vi "Register by Name.vi"(7 "Event":refnum<class "Event.lvclass">, 8 "error in (no error)":errorcluster, 9 "Event Fire Handler":refnum<class "Event Generated Msg.lvclass">, 10 "Sink Name":string, 11 "Event Source in":refnum<class "Event Source.lvclass">) -> (0 "error out":errorcluster, 3 "Event Source out":refnum<class "Event Source.lvclass">)   [LabVIEW 2016, in "Event Source.lvlib" / "Event Source.lvclass"]
uses:
  Event Source.lvclass
  Event/Event.lvclass
  Event Source Messages/Event Generated Msg/Event Generated Msg.lvclass
  Event Source.lvclass/Event Source.ctl
  <vilib>/ActorFramework/Message Enqueuer/Message Enqueuer.lvclass
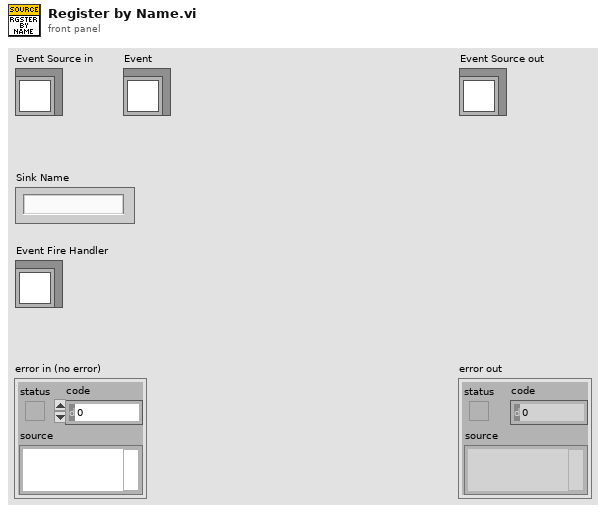
[diagram p1: front panel]
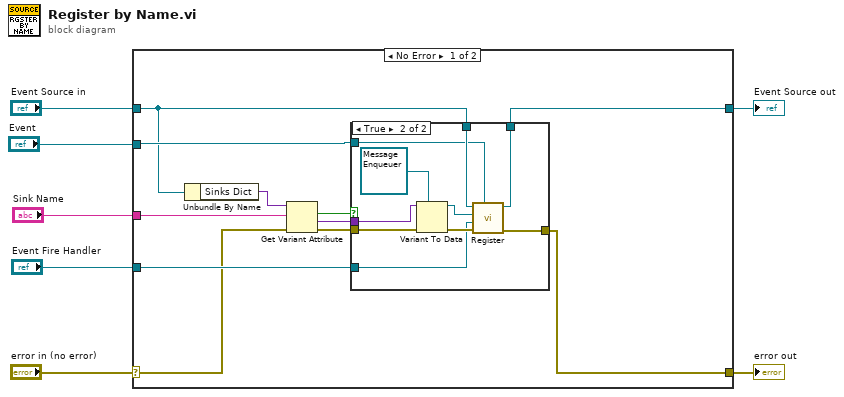
[diagram p0: block diagram]
diagram:
  n1 = case shown="No Error" "error in (no error)" {
    selector: "error in (no error)" -> [w9 w32]
    tunnel: [w8 w32] -> w6
    tunnel: [w10 w31] -> w4
    tunnel: "Event Source in" -> [w11 w31]
    tunnel: "Sink Name" -> [w17 _]
    tunnel: "Event Fire Handler" -> [w13 _]
    tunnel: "Event" -> [w12 _]
    frame No Error {
      n2 = Unbundle By Name(w11) -> ("Sinks Dict"=w18:variant)
      n3 = Get Variant Attribute(Variant=w18, name=w17, error in=w9) -> (found=w16:bool, value=w15:variant, error out=w14:errorcluster)  [unwired: 1 in, 1 out]
      n4 = case shown="True" w16 {
        tunnel: w15 -> [_ w28]
        tunnel: w14 -> [w20 w29]
        tunnel: w13 -> [_ w25]
        tunnel: w11 -> [w19 w24]
        tunnel: w12 -> [_ w23]
        tunnel: [w20 w22] -> w8
        tunnel: [w19 w21] -> w10
        frame False {
        }
        frame True {
          n5 = Variant To Data(error in=w29, type=refnum<class "Message Enqueuer.lvclass"> refnum ("Actor's Enqueuer"), Variant=w28) -> (data=w26:refnum<class "Message Enqueuer.lvclass">, error out=w27:errorcluster)
          n6 = call "Register.vi"("Event"=w23, "Error In"=w27, "Event Fire Handler"=w25, "Registrant Enq"=w26, "Event Source In"=w24) -> ("Error Out"=w22:errorcluster, "Event Source Out"=w21:refnum<class "Event Source.lvclass">)  [unwired: 5 in]
        }
      }
    }
    frame Error {
    }
  }
  "error out" <- w6
  "Event Source out" <- w4
